vi "Do.vi"(8 "error in (no error)":errorcluster, 10 "Actor in":refnum<class "Actor.lvclass">, 11 "Addition Request Msg":refnum<class "Addition Request Msg.lvclass">) -> (0 "error out":errorcluster, 2 "Actor out":refnum<class "Actor.lvclass">)   [LabVIEW 2014, in "Addition Request Msg.lvclass"]
doc: "(<B>Filename</B>: Actor Framework.lvlib:Message.lvclass:Do.vi)\n\nDefines what a message does when it is received by an actor. Generally, a message instructs an actor to invoke one of its methods. By default, this method does nothing. A child class must override it to define behavior. Create a child class by using the Actor Framework Message Maker dialog box."
uses:
  Addition Request Msg.lvclass
  <vilib>/ActorFramework/Actor/Actor.lvclass
  Addition Actor Class/Addition Actor.lvclass
  Addition Request Msg.lvclass/Addition Request Msg.ctl
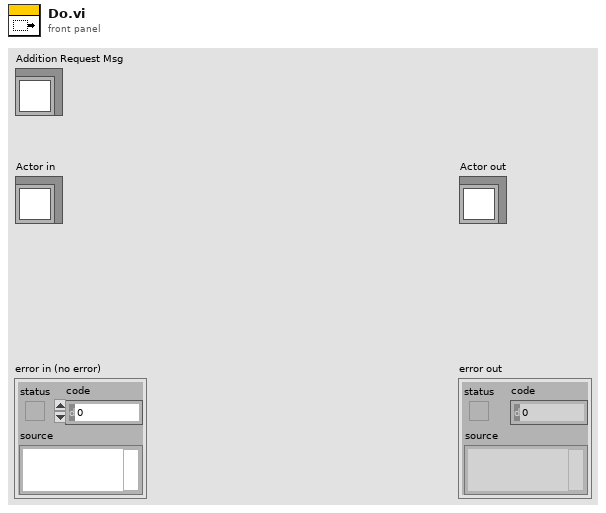
[diagram p1: front panel]
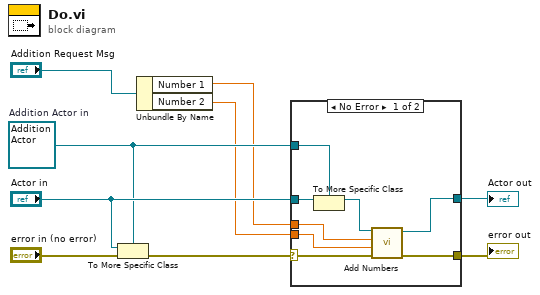
[diagram p0: block diagram]
diagram:
  w5 = refnum<class "Addition Actor.lvclass"> refnum  # Addition Actor in
  n1 = To More Specific Class(target class=w5, reference="Actor in", error in="error in (no error)") -> (error out=w7:errorcluster)  [unwired: 1 out]
  n2 = Unbundle By Name("Addition Request Msg") -> ("Number 1"=w2:dbl, "Number 2"=w1:dbl)
  n3 = case shown="No Error" w7 {
    selector: w7 -> [w16 w18]
    tunnel: "Actor in" -> [w17 w19]
    tunnel: [w15 w18] -> w6
    tunnel: w5 -> [w14 _]
    tunnel: [w12 w19] -> w4
    tunnel: w2 -> [w11 _]
    tunnel: w1 -> [w10 _]
    frame No Error {
      n4 = To More Specific Class(target class=w14, reference=w17) -> (specific class reference=w13:refnum<class "Addition Actor.lvclass">)  [unwired: 1 in, 1 out]
      n5 = call "Add Numbers.vi"("error in (no error)"=w16, "Number 2"=w10, "Number 1"=w11, "Addition Actor in"=w13) -> ("error out"=w15:errorcluster, "Addition Actor out"=w12:refnum<class "Addition Actor.lvclass">)  [unwired: 6 in]
    }
    frame Error {
    }
  }
  "error out" <- w6
  "Actor out" <- w4
